vi "LaunchDialog.vi"(7 "Queues":T1, 8 "error in (no error)":errorcluster, 10 "DialogData":variant, 11 "DialogPath":path) -> (0 "error out":errorcluster)   [LabVIEW 2017, in "Server.lvlib" / "Dialogs.lvlib"]
uses:
  Dialogs.lvlib
  Message Queue/CommReferences.ctl
  Message Queue/MessageCluster.ctl
  Message Queue/Message Queue.lvlib
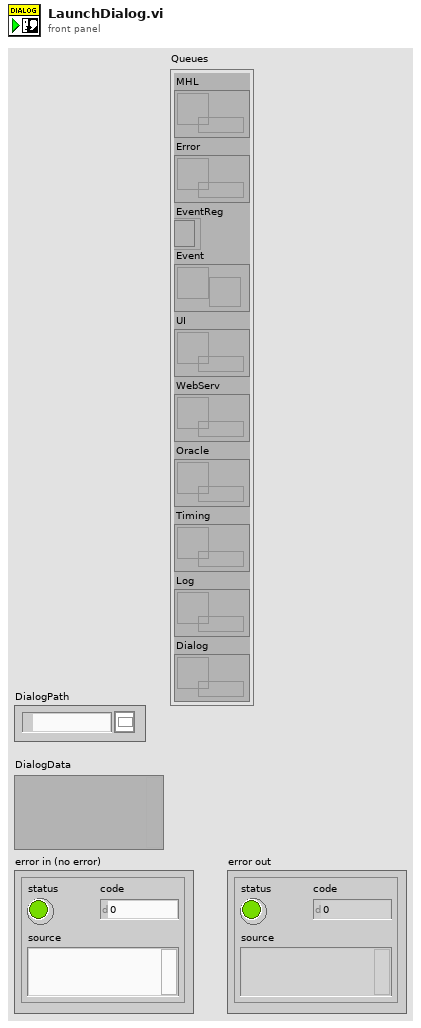
[diagram p1: front panel]
types:
  T1 = typedef "Server.lvlib/Message Queue.lvlib/CommReferences.ctl" = cluster{"MHL":refnum<queue>, "Error":refnum<queue>, "EventReg":refnum<event-registration>, "Event":refnum<user-event>, "UI":refnum<queue>, "WebServ":refnum<queue>, "Oracle":refnum<queue>, "Timing":refnum<queue>, "Log":refnum<queue>, "Dialog":refnum<queue>}
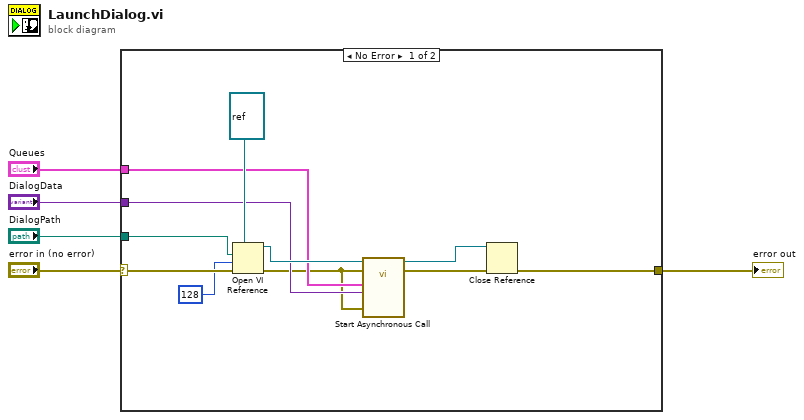
[diagram p0: block diagram]
diagram:
  n1 = case shown="No Error" "error in (no error)" {
    selector: "error in (no error)" -> [w15 w17]
    tunnel: "DialogPath" -> [w16 _]
    tunnel: [w12 w17] -> w4
    tunnel: "DialogData" -> [w8 _]
    tunnel: "Queues" -> [w7 _]
    frame No Error {
      n2 = Open VI Reference(type specifier VI Refnum (for type only)=refnum<vi> refnum, vi path=w16, options=128, error in (no error)=w15) -> (vi reference=w11:refnum<vi>, error out=w6:errorcluster)  [unwired: 2 in]
      n3 = call-by-ref "Start Asynchronous Call"(reference=w11, error in=w6, "Error In"=w6, "Data"=w8, "Queues"=w7) -> (reference out=w10:refnum<vi>, error out=w13:errorcluster)  [unwired: 9 in]
      n4 = Close Reference(reference=w10, error in (no error)=w13) -> (error out=w12:errorcluster)
    }
    frame Error {
    }
  }
  "error out" <- w4
